vi "Errorx.Set-Change Error Info.vi"(7 "Append Details":bool=TRUE, 8 "error in":errorcluster, 9 "Description":string, 10 "Code(0 = no change)":i32, 11 "Error Status":bool=TRUE) -> (0 "error out":errorcluster)   [LabVIEW 2024, in "EQMF.lvlib" / "Event Log.lvlib"]
uses:
  Event Log.lvlib
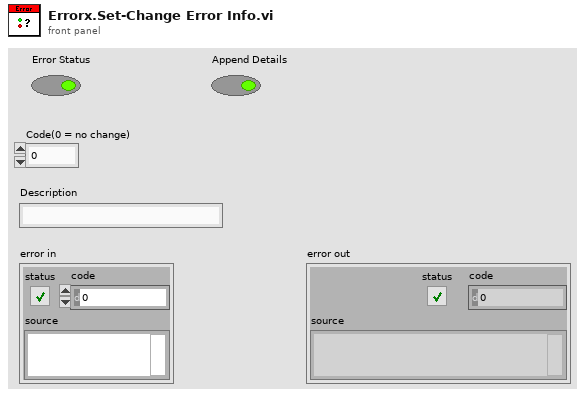
[diagram p1: front panel]
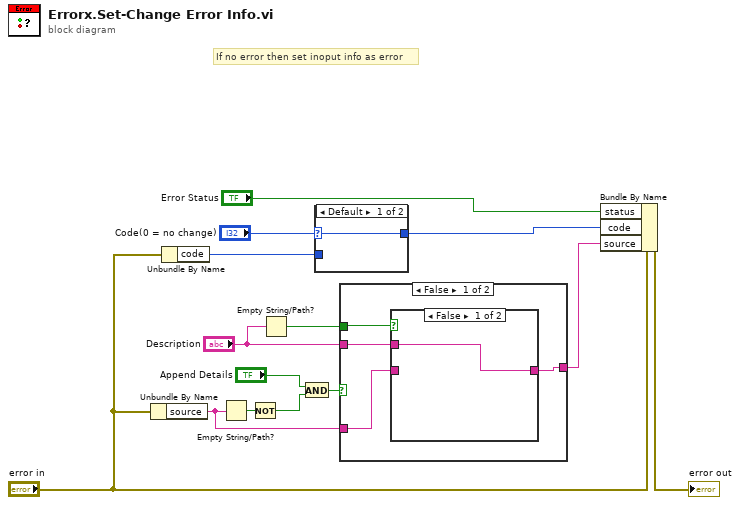
[diagram p0: block diagram]
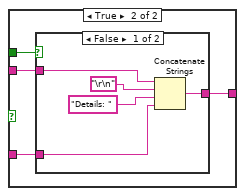
[diagram p4: hidden frame]
diagram:
  # "If no error then set inoput info as error"
  n1 = Unbundle By Name("error in") -> ("source"=w3:string)
  n2 = Unbundle By Name("error in") -> ("code"=w4:i32)
  n3 = Empty String/Path?(string/path=w3) -> (empty?=w12:bool)
  n4 = Not(x=w12) -> (.not. x?=w10:bool)
  n5 = Empty String/Path?(string/path="Description") -> (empty?=w1:bool)
  n6 = And(x="Append Details", y=w10) -> (x .and. y?=w8:bool)
  n7 = case shown="Default" "Code(0 = no change)" {
    selector: "Code(0 = no change)" -> [w15 _]
    tunnel: [w15 w16] -> w6
    tunnel: w4 -> [_ w16]
    frame Default {
    }
    frame 0 {
    }
  }
  n8 = case shown="False" w8 {
    tunnel: "Description" -> [w17 w26]
    tunnel: [w19 w25] -> w9
    tunnel: w3 -> [w18 w24]
    tunnel: w1 -> [w20 w23]
    frame False {
      n9 = case shown="False" w20 {
        tunnel: [w21 w22] -> w19
        tunnel: w18 -> [_ w22]
        tunnel: w17 -> [w21 _]
        frame False {
        }
        frame True {
        }
      }
    }
    frame True {
      n10 = case shown="False" w23 {
        tunnel: w26 -> [w29 _]
        tunnel: [w28 w32] -> w25
        tunnel: w24 -> [w27 w32]
        frame False {
          n11 = Concatenate Strings(w29, "\r\n", "Details: ", w27) -> (w28:string)
        }
        frame True {
        }
      }
    }
  }
  n12 = Bundle By Name(cluster="error in", "status"="Error Status", "code"=w6, "source"=w9) -> (→"error out":errorcluster)
